vi "Set Trace.vi"(8 "Error In":errorcluster, 10 "Trace":i32, 11 "Pixel In":refnum<class "Pixel.lvclass">) -> (0 "Error Out":errorcluster, 3 "Pixel Out":refnum<class "Pixel.lvclass">)   [LabVIEW 2019, in "Pixel.lvclass"]
uses:
  Pixel.lvclass
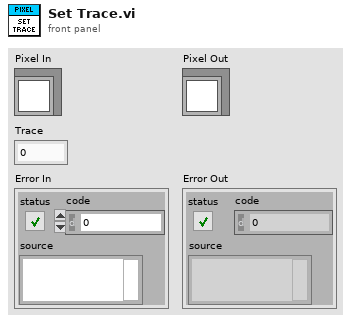
[diagram p1: front panel]
types:
  T1 = typedef "Pixel.lvclass/Data.ctl" = cluster{"Trace":i32, "Positions History":T2[]}
  T2 = typedef "Display Element.lvclass/Vector.ctl" = cluster{"X":i32, "Y":i32}
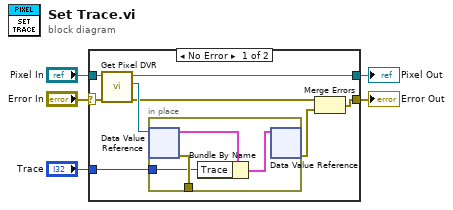
[diagram p0: block diagram]
diagram:
  n1 = case shown="No Error" "Error In" {
    selector: "Error In" -> [w10 w18]
    tunnel: [w12 w18] -> w4
    tunnel: [w7 w19] -> w1
    tunnel: "Pixel In" -> [w9 w19]
    tunnel: "Trace" -> [w11 _]
    frame No Error {
      n2 = call "Get Pixel DVR.vi"("Error In"=w10, "Pixel In"=w9) -> ("Error Out"=w6:errorcluster, "DVR"=w8:refnum<data-value>, "Pixel Out"=w7:refnum<class "Pixel.lvclass">)  [unwired: 7 in]
      n3 = in-place {
        in-place-border: [w17] -> _
        in-place-border: w11 -> [w14]
        n4 = in-place-dvr #1(w8) -> (w16:T1, w17:errorcluster)
        n5 = Bundle By Name(cluster=w16, "Trace"=w14) -> (w15:T1)
        n6 = in-place-dvr #1(w15) -> (w13:errorcluster)  [unwired: 1 out]
      }
      n7 = Merge Errors(w6, w13) -> (w12:errorcluster)
    }
    frame Error {
    }
  }
  "Pixel Out" <- w1
  "Error Out" <- w4
